vi "Set3dPos.vi"(1 "Index Type (Absolute)":T1=1 items=["Incremental", "Absolute", "Registration", "Jog"], 5 "Index (0)":T2, 7 "Position (mm)":T4, 11 "error in (no error)":errorcluster, 12 "Axis Settings":T3=[{"Velocity"=5.0, "Accel. / Decel."=5.0, "Dwell"=0}, {"Velocity"=5.0, "Accel. / Decel."=5.0, "Dwell"=0}, {"Velocity"=5.0, "Accel. / Decel."=5.0, "Dwell"=0}]) -> (6 "Index (duplicate)":T2, 15 "error out":errorcluster)   [LabVIEW 2009]
uses:
  typedefs/Position3d.ctl
  typedefs/AxesTestSettings.ctl
  typedefs/Ultra3000/Index_Numeric.ctl
  typedefs/Ultra3000/IndexType.ctl
  typedefs/Ultra3000/IndexSettings_Cluster.ctl
  typedefs/DwellTime.ctl
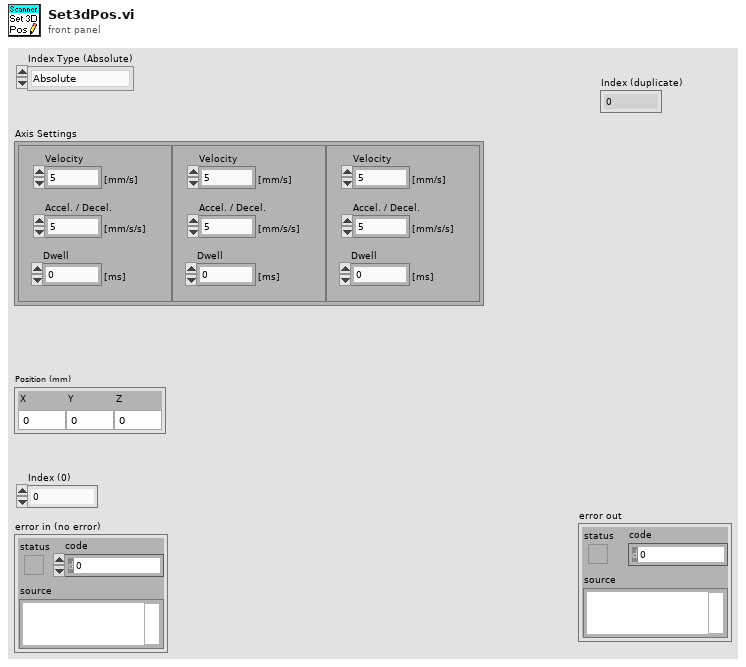
[diagram p1: front panel]
types:
  T1 = typedef "IndexType.ctl" = i32
  T2 = typedef "Index_Numeric.ctl" = u8
  T3 = typedef "AxesTestSettings.ctl" = cluster{"Velocity":dbl, "Accel. / Decel.":dbl, "Dwell":u16}[]
  T4 = typedef "Position3d.ctl" = cluster{"X":dbl, "Y":dbl, "Z":dbl}
  T5 = typedef "IndexSettings_Cluster.ctl" = cluster{"Type":T1, "Dwell":T6, "Velocity":dbl, "Accel/Decel":dbl}
  T6 = typedef "DwellTime.ctl" = u16
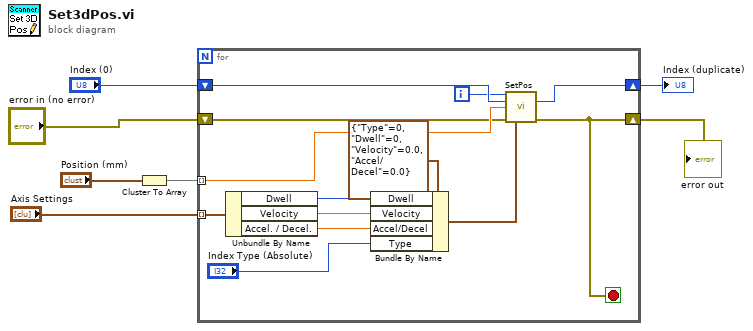
[diagram p0: block diagram]
diagram:
  n1 = Cluster To Array(cluster="Position (mm)") -> (array=w7:dbl[])
  n2 = for {
    tunnel: w7 -> [w11] mode=indexing
    tunnel: "Axis Settings" -> [w20] mode=indexing
    shift-right: [w15] -> w3
    shift-left: "Index (0)" -> [w16]
    shift-right: [w9] -> w1
    shift-left: "error in (no error)" -> [w8]
    i -> [w10]
    stop <- w9 stop-if-true
    n3 = Unbundle By Name(w20) -> ("Dwell"=w17:u16, "Velocity"=w19:dbl, "Accel. / Decel."=w18:dbl)
    n4 = Bundle By Name(cluster=T5 {"Type"=0, "Dwell"=0, "Velocity"=0.0, "Accel/Decel"=0.0} ("Index Settings"), "Dwell"=w17, "Velocity"=w19, "Accel/Decel"=w18, "Type"="Index Type (Absolute)") -> (w12:T5)
    n5 = call "SetPos.vi"("Axis In"=w10, "Index (0)"=w16, "Position"=w11, "error in (no error)"=w8, "Index Settings"=w12) -> ("Index (duplicate)"=w15:T2, "error out"=w9:errorcluster)  [unwired: 8 in, 1 out]
  }
  "Index (duplicate)" <- w3
  "error out" <- w1
